vi "calculate_deviation_from_spatial_standard.vi"(0 "Image Src":T1, 1 "Background Image":T1, 3 "error in (no error)":errorcluster) -> (6 "Processed Image":T1(plugin-control), 7 "transformation_description":dbl[](array[numeric]), 8 "fit least squares error (camera pixel)":dbl, 9 "max spatial drift (mm)":dbl, 10 "error out":errorcluster)   [LabVIEW 2019]
uses:
  <vilib>/vision/Image Controls.llb/IMAQ Image.ctl
  <vilib>/vision/Calibration.llb/Distortion Model.ctl
  <vilib>/vision/Calibration.llb/Distortion Model Types.ctl
  <vilib>/vision/Image Controls.llb/Vision Info Type2.ctl
  <vilib>/vision/Calibration.llb/Calibration Reference Points.ctl
  ParametersGlobal.vi
  DebugGlobal.vi
  <vilib>/vision/NI_Vision_Development_Module.lvlib
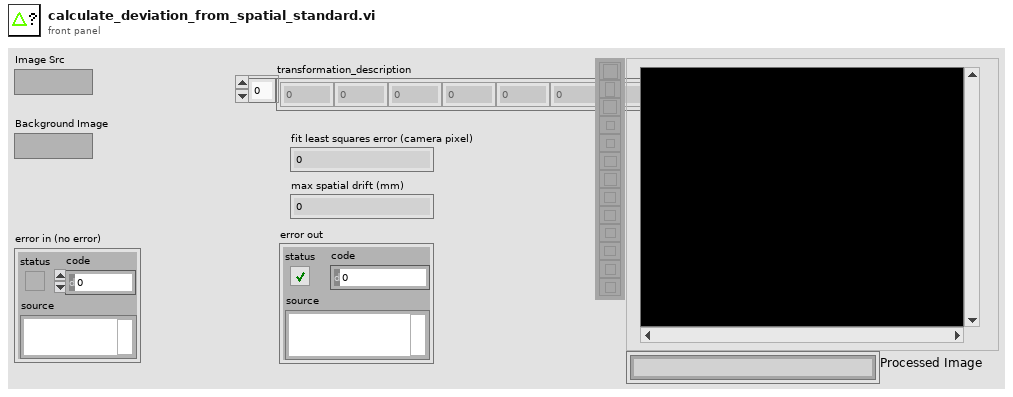
[diagram p1: front panel]
types:
  T1 = typedef "IMAQ Image.ctl" = refnum<image>
  T2 = typedef "Image Type" = u32
  T3 = typedef "Calibration Reference Points.ctl" = cluster{"Pixel Coordinates":cluster{"X":dbl, "Y":dbl}[], "Real World Coordinates":cluster{"X":dbl, "Y":dbl}[], "Unit":T4, "Image Size":cluster{"X":u32, "Y":u32}}
  T4 = typedef "Image Unit" = enum32{"Undefined", "Angström", "Micrometer", "Millimeter", "Centimeter", "Meter", "Kilometer", "Microinch", "Inch", "Feet", "Nautical miles", "Standard miles", "Steps"}
  T5 = typedef "Vision Info Type2.ctl" = u32
  T6 = typedef "Distortion Model.ctl" = cluster{"Distortion Model":T7, "Polynomial Model Setup":cluster{"Radial Coefficient":u32, "Tangential Coefficients ":bool}}
  T7 = typedef "Distortion Model Types.ctl" = i32
  T8 = cluster{"Left":i32, "Top":i32, "Right":i32, "Bottom":i32}
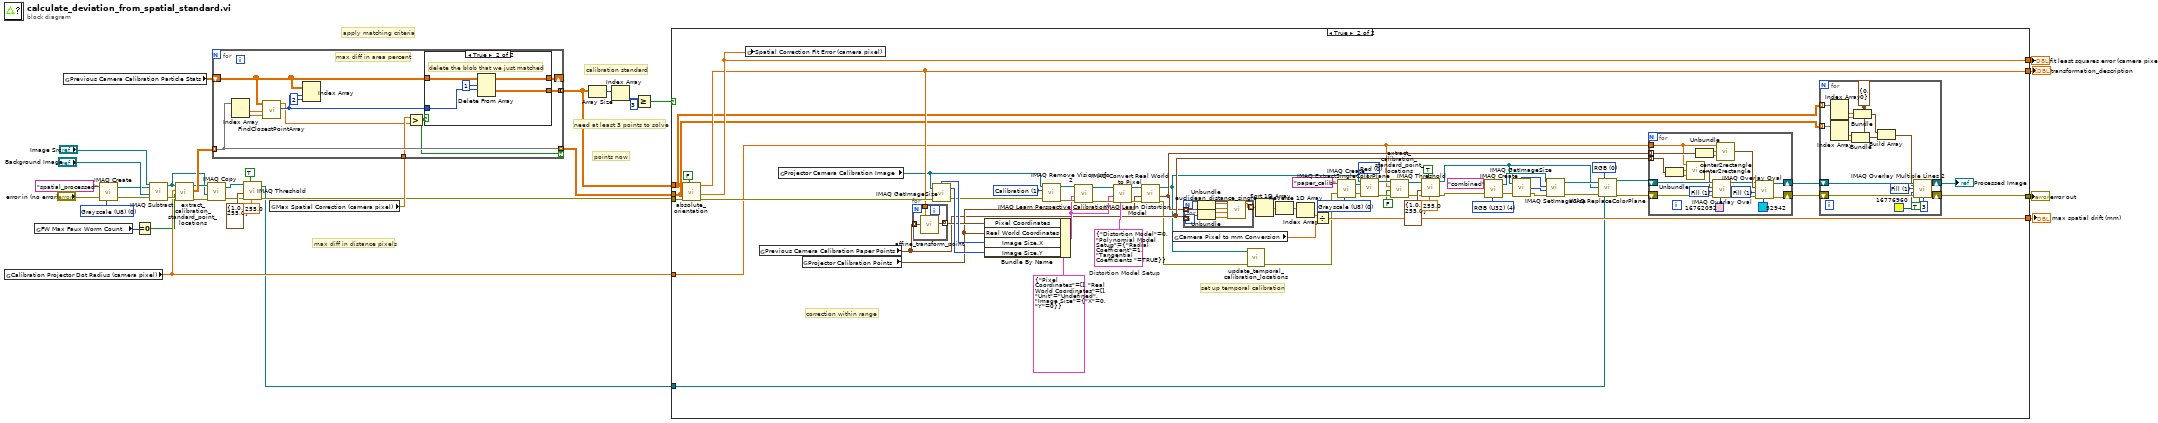
[diagram p0: block diagram]
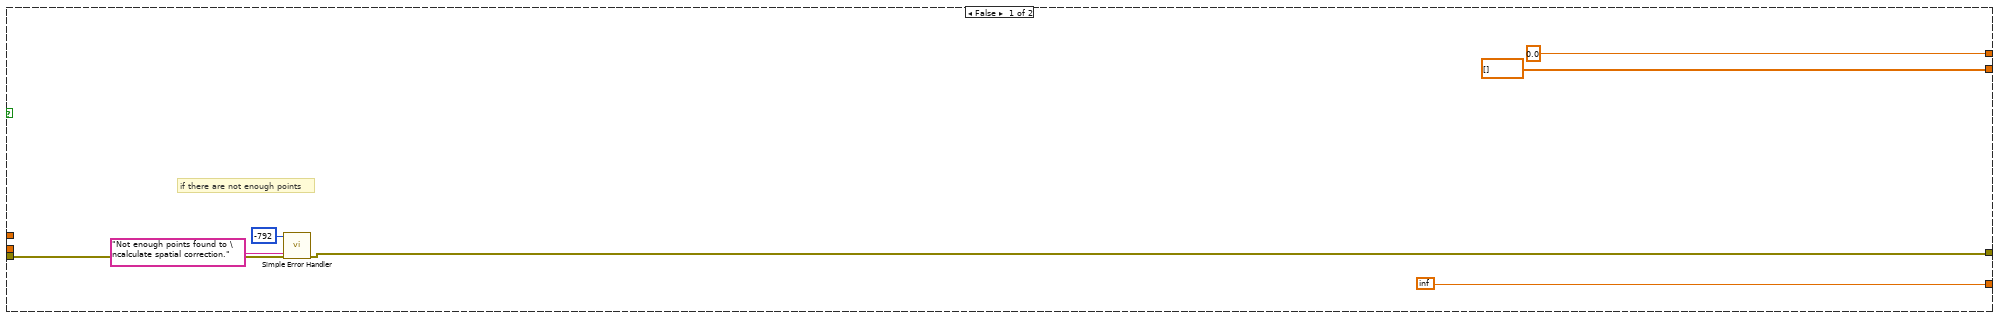
[diagram p2: hidden frame]
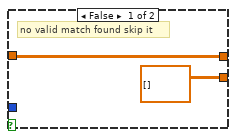
[diagram p3: hidden frame]
diagram:
  w23 = T2 0 items=["Grayscale (U8)", "Grayscale (I16)", "Grayscale (SGL)", "Complex (CSG)", "RGB (U32)", "HSL (U32)", "RGB (U64)", "Grayscale (U16)"] ("Image Type")
  # "need at least 3 points to solve"
  # "points now"
  # "calibration standard"
  # "max diff in distance pixels"
  # "apply matching criteria"
  n1 = global read "ParametersGlobal.vi" "Calibration Projector Dot Radius (camera pixel)"() -> (w13:dbl)
  n2 = global read "ParametersGlobal.vi" "FW Max Faux Worm Count"() -> (w10:i32)
  n3 = global read "ParametersGlobal.vi" "Previous Camera Calibration Particle Stats"() -> (w34:dbl[][])
  n4 = call "IMAQ Create"("Image Name"="spatial_processed", "Image Type"=w23, "error in (no error)"="error in (no error)") -> ("New Image"=w25:T1, "error out"=w26:errorcluster)  [unwired: 2 in]
  n5 = Equal To 0?(x=w10) -> (x = 0?=w9:bool)
  n6 = call "IMAQ Subtract"("Image Src A"="Image Src", "Image Dst"=w25, "Image Src B"="Background Image", "error in (no error)"=w26) -> ("Image Dst Out"=w2:T1, "error out"=w28:errorcluster)  [unwired: 3 in]
  n7 = call "extract_calibration_standard_point_locations.vi"("error in (no error)"=w28, "Agar (T) Paper (F)"=w9, "expected dot radius (camera pixels)"=w13, "Image Src"=w2) -> ("error out"=w5:errorcluster, "Particle Measurements (Pixels)"=w16:dbl[][], "Image Out (duplicate)"=w3:T1)  [unwired: 5 in]
  n8 = call "IMAQ Copy"("error in (no error)"=w5, "Image Dst"=w2, "Image Src"=w3) -> ("error out"=w4:errorcluster, "Image Dst Out"=w1:T1)  [unwired: 3 in]
  n9 = call "IMAQ Threshold"("Replace Value"=sgl 255.0, "Keep/Replace Value (Replace)"=TRUE, "error in (no error)"=w4, "Range"=cluster{"Lower value":sgl, "Upper value":sgl} {"Lower value"=1.0, "Upper value"=255.0}, "Image Src"=w1) -> ("error out"=w12:errorcluster, "Image Dst Out"=w11:T1)  [unwired: 5 in]
  n10 = global read "ParametersGlobal.vi" "Max Spatial Correction (camera pixel)"() -> (w22:dbl)
  n11 = for {
    shift-right: [w45] -> _
    shift-left: w34 -> [w40]
    tunnel: w16 -> [w41] mode=indexing
    tunnel: [w42] -> w21 mode=concatenating
    tunnel: [w41] -> w33 mode=indexing if=w35
    tunnel: w22 -> [w37]
    # "max diff in area percent"
    n12 = Index Array(array=w41) -> (element #1=w44:dbl, element #2=w43:dbl)  [unwired: 2 in]
    n13 = call "FindClosestPointArray.vi"("Y"=w43, "X"=w44, "Particle Measurements (Pixels)"=w40) -> ("ShortestDistanceIndex"=w39:i32, "ShortestDistance"=w36:sgl)  [unwired: 7 in]
    n14 = Index Array(array=w40, index (row)=w39, index (col)=2 ("disabled index (col)")) -> ()  [unwired: 1 out]
    n15 = Greater?(x=w37, y=w36) -> (0:w35:bool)
    n16 = case shown="True" w35 {
      tunnel: w40 -> [w47 w52]
      tunnel: [w47 w50] -> w45
      tunnel: w39 -> [_ w49]
      tunnel: [dbl[][] [] ("Spatial Calibration Standard Points") w48] -> w42
      frame False {
        # "no valid match found skip it"
      }
      frame True {
        # "delete the blob that we just matched"
        n17 = Delete From Array(array=w52, length=1, index (row)=w49) -> (deleted portion=w48:dbl[][], array with subset deleted=w50:dbl[][])  [unwired: 1 in]
      }
    }
  }
  n18 = Array Size(array=w21) -> (size(s)=w20:i32[])
  n19 = Index Array(array=w20) -> (element=w19:i32)  [unwired: 1 in]
  n20 = Greater Or Equal?(x=w19, y=3) -> (x >= y?=w17:bool)
  n21 = case shown="True" w17 {
    tunnel: w33 -> [_ w119]
    tunnel: w12 -> [w59 w126]
    tunnel: [0.0 ("least squares error") w124] -> w32
    tunnel: [dbl[] [] ("transformation_description") w122] -> w31
    tunnel: w21 -> [_ w118]
    tunnel: [inf w121] -> w15
    tunnel: w11 -> [_ w63]
    tunnel: [w53 w120] -> w14
    tunnel: w13 -> [_ w80]
    frame False {
      # "if there are not enough points"
      n22 = call <vilib>:"Simple Error Handler.vi"("error code (no error:0)"=-792, "error source (\" \")"="Not enough points found to \ncalculate spatial correction." ("error source (\" \")"), "error in (no error)"=w59) -> ("error out"=w53:errorcluster)  [unwired: 2 in, 4 out]
    }
    frame True {
      w66 = u16 0 items=["RGB", "HSL", "HSV", "HSI"] ("Color Mode")
      w68 = T2 4 items=["Grayscale (U8)", "Grayscale (I16)", "Grayscale (SGL)", "Complex (CSG)", "RGB (U32)", "HSL (U32)", "RGB (U64)", "Grayscale (U16)"] ("Image Type")
      w84 = T2 0 items=["Grayscale (U8)", "Grayscale (I16)", "Grayscale (SGL)", "Complex (CSG)", "RGB (U32)", "HSL (U32)", "RGB (U64)", "Grayscale (U16)"] ("Image Type")
      w88 = 0 items=["Red", "Green", "Blue", "Hue", "Saturation", "Luminance", "Value", "Intensity"] ("Color Plane")
      w112 = T5 1 items=["Any", "Calibration", "Overlay", "Grayscale Template", "Color Template", "Geometric Template", "Custom Data", "Golden Template", "Geometric Template 2", "Contour Data", "Camera Model", "Pyramid Grayvalue Template", "Pyramid Gradient Template"] ("Vision Info")
      w115 = T6 {"Distortion Model"=0, "Polynomial Model Setup"={"Radial Coefficient"=1, "Tangential Coefficients "=TRUE}}  # Distortion Model Setup
      # "set up temporal calibration"
      # "correction within range"
      n23 = call "absolute_orientation.vi"("doScale"=FALSE, "error in"=w126, "Mapped To"=w119, "Mapped From"=w118) -> ("error out"=w125:errorcluster, "least squares error"=w124:dbl, "transformation_description"=w122:dbl[])  [unwired: 5 in]
      n24 = global write "DebugGlobal.vi" "Spatial Correction Fit Error (camera pixel)"(w124) -> ()
      n25 = global read "ParametersGlobal.vi" "Previous Camera Calibration Paper Points"() -> (w101:cluster{"X":dbl, "Y":dbl}[])
      n26 = global read "ParametersGlobal.vi" "Projector Camera Calibration Image"() -> (w102:T1)
      n27 = global read "ParametersGlobal.vi" "Projector Calibration Points"() -> (w103:cluster{"X":dbl, "Y":dbl}[])
      n28 = for {
        tunnel: w122 -> [w173]
        tunnel: [w172] -> w104 mode=indexing
        tunnel: w101 -> [w171] mode=indexing
        n29 = call "affine_transform_point.vi"("Pixel Coordinates In"=w171, "transformation_description"=w173) -> ("Pixel Coordinates Out"=w172:cluster{"X":sgl, "Y":sgl})  [unwired: 9 in]
      }
      n30 = call "IMAQ GetImageSize"("Image"=w102, "error in (no error)"=w125) -> ("Y Resolution"=w113:i32, "X Resolution"=w114:i32, "error out"=w111:errorcluster)  [unwired: 2 in]
      n31 = Bundle By Name(cluster=T3 {"Pixel Coordinates"=[], "Real World Coordinates"=[], "Unit"=enum."Undefined", "Image Size"={"X"=0, "Y"=0}} ("Reference Points"), "Pixel Coordinates"=w104, "Real World Coordinates"=w103, "Image Size.X"=w114, "Image Size.Y"=w113) -> (w108:T3)
      n32 = call "IMAQ Remove Vision Info 2"("error in (no error)"=w111, "Vision Info"=w112, "Image"=w102) -> ("error out"=w110:errorcluster, "Image Out"=w109:T1)  [unwired: 7 in]
      n33 = call "IMAQ Learn Perspective Calibration"("error in (no error)"=w110, "Reference Points"=w108, "Calibration Template Image"=w109) -> ("error out"=w117:errorcluster, "Calibration Template Image Out"=w116:T1)  [unwired: 1 in, 6 out]
      n34 = call "IMAQ Learn Distortion Model"("Distortion Model Setup"=w115, "error in (no error)"=w117, "Reference Points"=w108, "Calibration Template Image"=w116) -> ("error out"=w106:errorcluster, "Calibration Template Image Out"=w105:T1)  [unwired: 2 in, 4 out]
      n35 = call "IMAQ Convert Real World to Pixel"("error in (no error)"=w106, "Array of Real World Coordinates"=w103, "Calibrated Image"=w105) -> ("error out"=w99:errorcluster, "Array of Pixel Coordinates"=w100:cluster{"X":sgl, "Y":sgl}[], "Calibrated Image (duplicate)"=w86:T1)  [unwired: 3 in, 3 out]
      n36 = global read "ParametersGlobal.vi" "Camera Pixel to mm Conversion"() -> (w95:sgl)
      n37 = for {
        tunnel: w100 -> [w170] mode=indexing
        tunnel: w101 -> [w169] mode=indexing
        tunnel: [w164] -> w94 mode=indexing
        n38 = Unbundle(w170) -> ("X"=w165:sgl, "Y"=w166:sgl)
        n39 = Unbundle(w169) -> ("X"=w167:dbl, "Y"=w168:dbl)
        n40 = call "euclidean_distance_single.vi"("Point 2 Y"=w168, "Point 2 X"=w167, "Point 1 Y"=w166, "Point 1 X"=w165) -> ("Distance"=w164:sgl)  [unwired: 7 in]
      }
      n41 = call "update_temporal_calibration_locations.vi"("error in (no error)"=w99, "Projector to Camera Calibration in"=w86) -> ("error out"=w89:errorcluster)  [unwired: 9 in]
      n42 = Sort 1D Array(array=w94) -> (sorted array=w93:sgl[])
      n43 = Reverse 1D Array(array=w93) -> (reversed array=w92:sgl[])
      n44 = Index Array(array=w92) -> (element=w91:sgl)  [unwired: 1 in]
      n45 = Divide(x=w91, y=w95) -> (x/y=w121:sgl)
      n46 = call "IMAQ Create"("Image Name"="paper_calib", "Image Type"=w84, "error in (no error)"=w89) -> ("New Image"=w85:T1, "error out"=w87:errorcluster)  [unwired: 2 in]
      n47 = call "IMAQ ExtractSingleColorPlane"("Color Plane"=w88, "error in (no error)"=w87, "Image Dst"=w85, "Image Src"=w86) -> ("error out"=w83:errorcluster, "Image Dst Out"=w82:T1)  [unwired: 6 in]
      n48 = call "extract_calibration_standard_point_locations.vi"("error in (no error)"=w83, "Agar (T) Paper (F)"=FALSE, "expected dot radius (camera pixels)"=w80, "Image Src"=w82) -> ("error out"=w76:errorcluster, "Image Out (duplicate)"=w75:T1)  [unwired: 5 in, 1 out]
      n49 = call "IMAQ Threshold"("Replace Value"=sgl 255.0, "Keep/Replace Value (Replace)"=TRUE, "error in (no error)"=w76, "Range"=cluster{"Lower value":sgl, "Upper value":sgl} {"Lower value"=1.0, "Upper value"=255.0}, "Image Src"=w75) -> ("error out"=w69:errorcluster, "Image Dst Out"=w62:T1)  [unwired: 5 in]
      n50 = call "IMAQ Create"("Image Name"="combined", "Image Type"=w68, "error in (no error)"=w69) -> ("New Image"=w71:T1, "error out"=w70:errorcluster)  [unwired: 2 in]
      n51 = call "IMAQ GetImageSize"("Image"=w62, "error in (no error)"=w70) -> ("Y Resolution"=w73:i32, "X Resolution"=w72:i32, "error out"=w74:errorcluster)  [unwired: 2 in]
      n52 = call "IMAQ SetImageSize"("error in (no error)"=w74, "Y Resolution"=w73, "X Resolution"=w72, "Image"=w71) -> ("error out"=w65:errorcluster, "Image Out"=w64:T1)  [unwired: 1 in]
      n53 = call "IMAQ ReplaceColorPlane"("Image Src"=w64, "Color Mode"=w66, "Red or Hue Plane"=w62, "error in (no error)"=w65, "Blue or Luma or Val or Inten Plane"=w63) -> ("Image Dst Out"=w60:T1, "error out"=w61:errorcluster)  [unwired: 9 in]
      n54 = for {
        tunnel: w101 -> [w157] mode=indexing
        shift-right: [w148] -> w97
        shift-left: w60 -> [w161]
        shift-right: [w147] -> w98
        shift-left: w61 -> [w162]
        tunnel: w100 -> [w146] mode=indexing
        tunnel: w80 -> [w145]
        w150 = u32 1 items=["Frame", "Fill"] ("Drawing Mode (Frame)")
        w158 = u32 1 items=["Frame", "Fill"] ("Drawing Mode (Frame)")
        n55 = Unbundle(w157) -> ("X"=w156:dbl, "Y"=w155:dbl)
        n56 = call "center2rectangle.vi"("Center Y"=w155, "Center X"=w156, "Box Half Size"=w145) -> ("Box Rectangle"=w154:T8)
        n57 = Unbundle(w146) -> ("X"=w153:sgl, "Y"=w152:sgl)
        n58 = call "IMAQ Overlay Oval"("Color"=u32 16762052, "error in (no error)"=w162, "Drawing Mode (Frame)"=w158, "Bounding Rectangle"=w154, "Image"=w161) -> ("error out"=w159:errorcluster, "Image Out"=w149:T1)  [unwired: 5 in]
        n59 = call "center2rectangle.vi"("Center Y"=w152, "Center X"=w153, "Box Half Size"=w145) -> ("Box Rectangle"=w151:T8)
        n60 = call "IMAQ Overlay Oval"("Color"=u32 52942, "error in (no error)"=w159, "Drawing Mode (Frame)"=w150, "Bounding Rectangle"=w151, "Image"=w149) -> ("error out"=w147:errorcluster, "Image Out"=w148:T1)  [unwired: 5 in]
      }
      n61 = for {
        shift-right: [w142] -> w96
        shift-left: w97 -> [w141]
        shift-right: [w143] -> w120
        shift-left: w98 -> [w144]
        tunnel: w119 -> [w137] mode=indexing
        tunnel: w118 -> [w140] mode=indexing
        w130 = u32 1 items=["Frame", "Fill"] ("Drawing Mode (Frame)")
        w135 = cluster{"X":i32, "Y":i32} {"X"=0, "Y"=0} ("Start Point")
        n62 = Index Array(array=w140) -> (element #1=w139:dbl, element #2=w138:dbl)  [unwired: 2 in]
        n63 = Index Array(array=w137) -> (element #1=w136:dbl, element #2=w134:dbl)  [unwired: 2 in]
        n64 = Bundle(cluster=w135, "X"=w136, "Y"=w134) -> (w133:cluster{"X":i32, "Y":i32})
        n65 = Bundle(cluster=w135, "X"=w139, "Y"=w138) -> (w132:cluster{"X":i32, "Y":i32})
        n66 = Build Array(w132, w133) -> (w129:cluster{"X":i32, "Y":i32}[])
        n67 = call "IMAQ Overlay Multiple Lines 2"("Image"=w141, "Line End Points"=w129, "Drawing Mode (Frame)"=w130, "Color"=u32 16776960, "error in (no error)"=w144, "Maintain Width?"=TRUE, "Width"=u32 3) -> ("Image Out"=w142:T1, "error out"=w143:errorcluster)  [unwired: 7 in]
      }
      "Processed Image" <- w96
    }
  }
  "fit least squares error (camera pixel)" <- w32
  "transformation_description" <- w31
  "max spatial drift (mm)" <- w15
  "error out" <- w14
